vi "Leja Order Roots (CDB).vi"(11 "Roots":cdb[](array[numeric])) -> (3 "Roots of Leja Order":cdb[](array[numeric]))   [LabVIEW 2020, in "NI_AALPro.lvlib"]
uses:
  NI_AALPro.lvlib
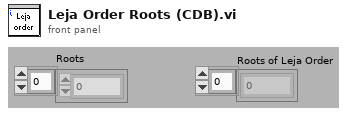
[diagram p1: front panel]
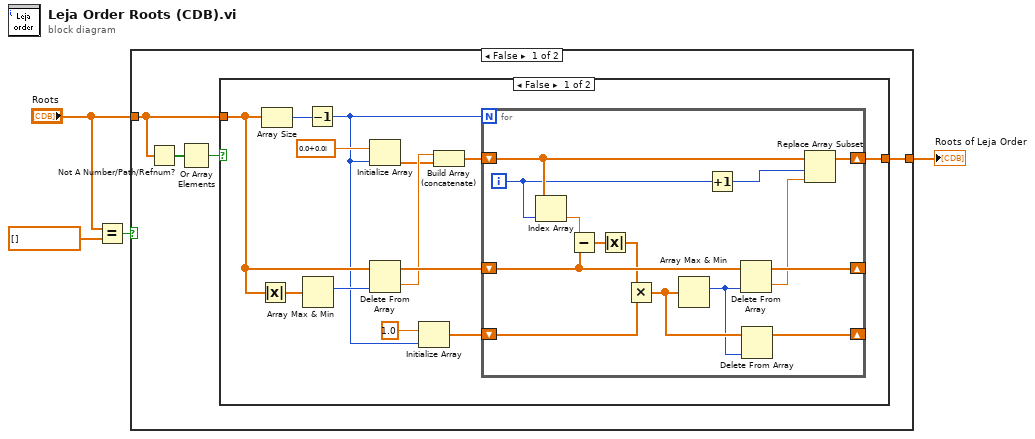
[diagram p0: block diagram]
diagram:
  n1 = Equal?(x="Roots", y=cdb[] []) -> (x = y?=w1:bool)
  n2 = case shown="False" w1 {
    tunnel: "Roots" -> [w7 _]
    tunnel: [w8 _] -> w4
    frame False {
      n3 = Not A Number/Path/Refnum?(number/path/refnum=w7) -> (NaN/Path/Refnum?=w6:bool[])
      n4 = Or Array Elements(Boolean array=w6) -> (logical OR=w5:bool)
      n5 = case shown="False" w5 {
        tunnel: w7 -> [w20 w36]
        tunnel: [w15 w36] -> w8
        frame False {
          n6 = Absolute Value(x=w20) -> (abs(x)=w21:dbl[])
          n7 = Array Size(array=w20) -> (size(s)=w17:i32)
          n8 = Array Max & Min(array=w21) -> (max index (indices)=w19:i32)  [unwired: 3 out]
          n9 = Decrement(x=w17) -> (x-1=w11:i32)
          n10 = Initialize Array(cdb 0.0+0.0i ("element"), w11) -> (w12:cdb[])
          n11 = Delete From Array(array=w20, index=w19) -> (deleted portion=w14:cdb, array with subset deleted=w18:cdb[])  [unwired: 1 in]
          n12 = Initialize Array(1.0, w11) -> (w9:dbl[])
          n13 = Build Array (concatenate)(w14, w12) -> (w16:cdb[])
          n14 = for {
            N: w11 -> [_]
            shift-right: [w34] -> w15
            shift-left: w16 -> [w31]
            shift-right: [w35] -> _
            shift-left: w18 -> [w29]
            shift-right: [w25] -> _
            shift-left: w9 -> [w22]
            i -> [w30]
            n15 = Index Array(array=w31, index=w30) -> (element=w28:cdb)
            n16 = Subtract(x=w28, y=w29) -> (x-y=w27:cdb[])
            n17 = Absolute Value(x=w27) -> (abs(x)=w23:dbl[])
            n18 = Multiply(x=w23, y=w22) -> (x*y=w26:dbl[])
            n19 = Array Max & Min(array=w26) -> (max index (indices)=w24:i32)  [unwired: 3 out]
            n20 = Increment(x=w30) -> (x+1=w32:i32)
            n21 = Delete From Array(array=w29, index=w24) -> (deleted portion=w33:cdb, array with subset deleted=w35:cdb[])  [unwired: 1 in]
            n22 = Delete From Array(array=w26, index=w24) -> (array with subset deleted=w25:dbl[])  [unwired: 1 in, 1 out]
            n23 = Replace Array Subset(array=w31, new element=w33, index=w32) -> (w34:cdb[])
          }
        }
        frame True {
        }
      }
    }
    frame True {
    }
  }
  "Roots of Leja Order" <- w4
